vi "gfitsio-error-cluster-from-code.vi"(8 "error in (no error)":errorcluster, 11 "error code":i32) -> (0 "error out":errorcluster)   [LabVIEW 2015]
doc: "Converts an error code to an error cluster. If the CFITSIO error stack contains messages, these are placed in the \"source\" field of <B>error out</B>. If <B>error in</B> indicates that an error occurred before this VI or function ran, <B>error out</B> contains the same error information. Otherwise, it describes the error status corresponding to the <B>error code</B>."
uses:
  gfitsio.dll
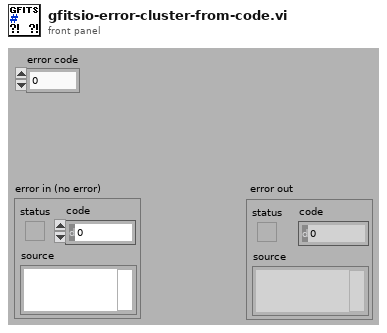
[diagram p1: front panel]
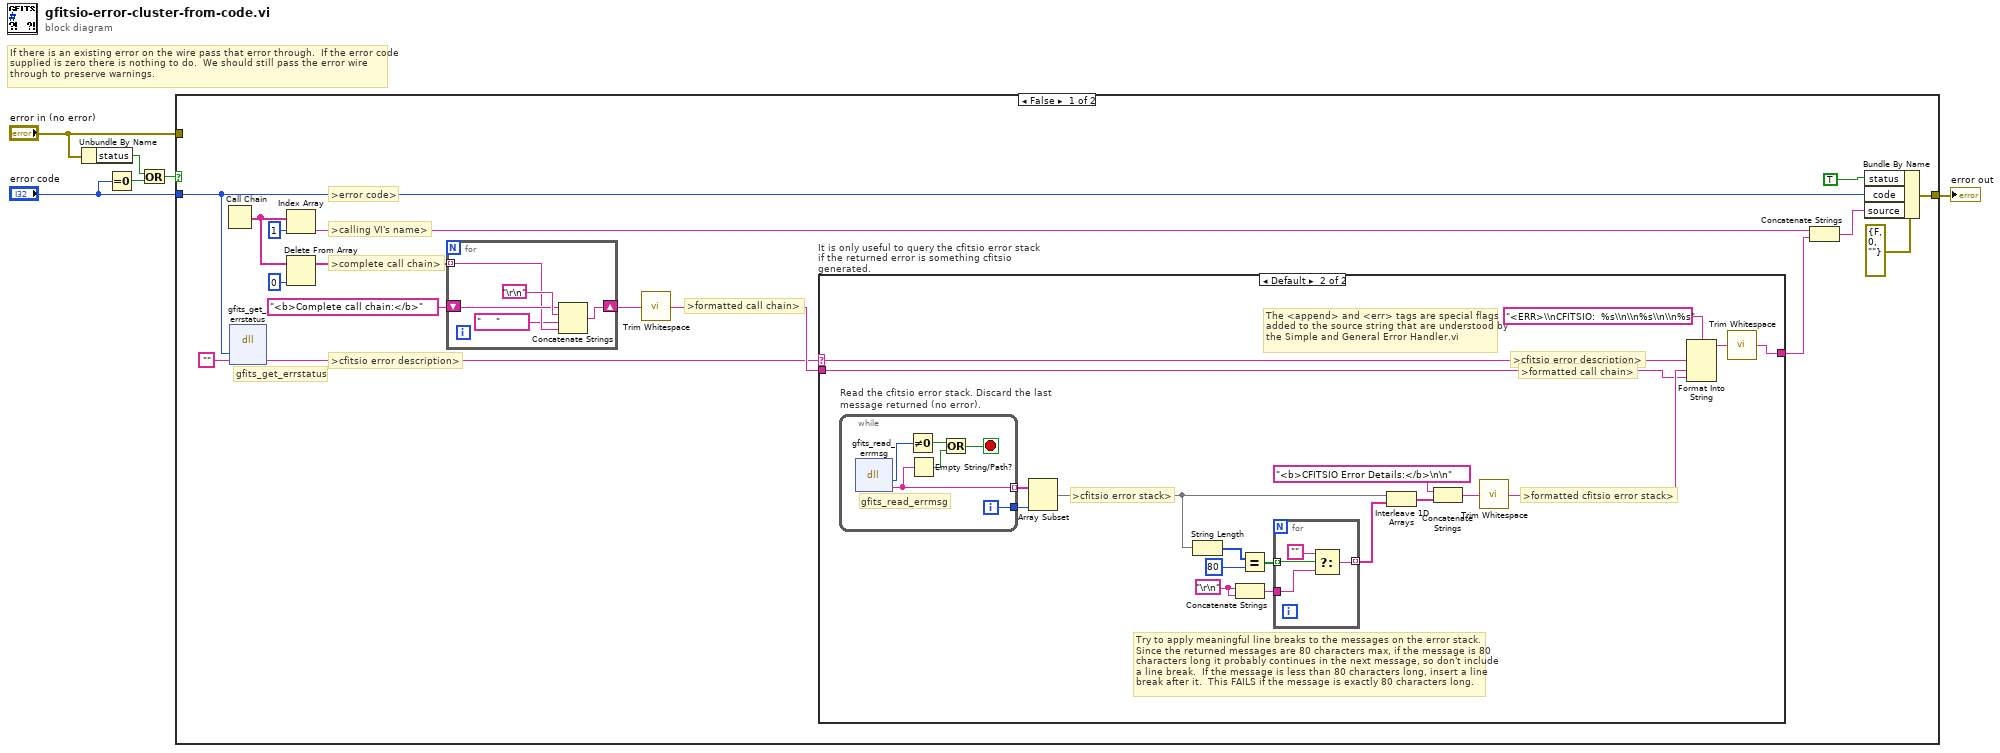
[diagram p0: block diagram]
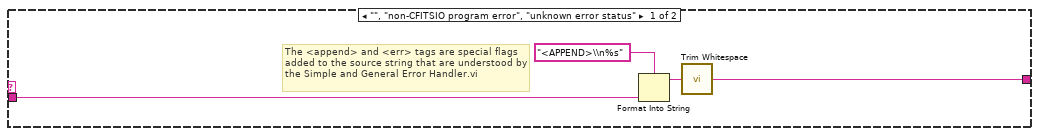
[diagram p2: hidden frame]
diagram:
  # "If there is an existing error on the wire pass that error through.  If the error code supplied is zero there is nothing to do.  We should still pass the error wire through to preserve warnings."
  n1 = Unbundle By Name("error in (no error)") -> ("status"=w4:bool)
  n2 = Equal To 0?(x="error code") -> (x = 0?=w5:bool)
  n3 = Or(x=w4, y=w5) -> (x .or. y?=w3:bool)
  n4 = case shown="False" w3 {
    tunnel: "error code" -> [w8 _]
    tunnel: "error in (no error)" -> [_ w60]
    tunnel: [w7 w60] -> w1
    frame False {
      # ">formatted call chain>"
      # ">cfitsio error description>"
      # "gfits_get_errstatus"
      # ">complete call chain>"
      # ">calling VI's name>"
      # ">error code>"
      n5 = Call Chain() -> (call chain=w18:string[])
      n6 = dll-call lib="C:/ALPHA GSCS/GSCS/Systems/SIcamera_Control/Quick_Look/gfitsio/gfitsio.dll" fn="gfits_get_errstatus"("status"=w8, "err_text"="") -> ("err_text"=w9:string)  [unwired: 5 in, 2 out]
      n7 = Index Array(array=w18, index=1) -> (element=w12:string)
      n8 = Delete From Array(array=w18, index=0) -> (array with subset deleted=w20:string[])  [unwired: 1 in, 1 out]
      n9 = for {
        tunnel: w20 -> [w56] mode=indexing
        shift-right: [w59] -> w11
        shift-left: "<b>Complete call chain:</b>" ("call chain header") -> [w57]
        n10 = Concatenate Strings(w57, "\r\n", "     ", w56) -> (w59:string)
      }
      n11 = call <vilib>:"Trim Whitespace.vi"("string"=w11) -> ("trimmed string"=w10:string)  [unwired: 1 in]
      n12 = case "It is only useful to query the cfitsio error stack if the returned error is something cfitsio generated." shown="Default" w9 {
        selector: w9 -> [_ w27]
        tunnel: [w24 w40] -> w13
        tunnel: w10 -> [w23 w28]
        frame "", "non-CFITSIO program error", "unknown error status" {
          # "The <append> and <err> tags are special flags added to the source string that are understood by the Simple and General Error Handler.vi"
          n13 = Format Into String(format string="<APPEND>\\n%s", w23) -> (resulting string=w26:string)  [unwired: 2 in, 1 out]
          n14 = call <vilib>:"Trim Whitespace.vi"("string"=w26) -> ("trimmed string"=w24:string)  [unwired: 1 in]
        }
        frame Default {
          w33 = "\r\n"
          # ">cfitsio error description>"
          # ">formatted call chain>"
          # "The <append> and <err> tags are special flags added to the source string that are understood by the Simple and General Error Handler.vi"
          # ">formatted cfitsio error stack>"
          # "Try to apply meaningful line breaks to the messages on the error stack.  Since the returned messages are 80 characters max, if the message is 80 characters long it probably continues in the next message, so don't include a line break.  If the message is less than 80 characters long, insert a line break after it.  This FAILS if the message is exactly 80 characters long."
          # ">cfitsio error stack>"
          n15 = while "Read the cfitsio error stack. Discard the last message returned (no error)." {
            tunnel: [w54] -> w44 mode=indexing
            tunnel: [w53] -> w43
            i -> [w53]
            stop <- w49 stop-if-true
            # "gfits_read_errmsg"
            n16 = dll-call lib="C:/ALPHA GSCS/GSCS/Systems/SIcamera_Control/Quick_Look/gfitsio/gfitsio.dll" fn="gfits_read_errmsg"() -> (w52:i32, "err_text"=w54:string)  [unwired: 4 in, 2 out]
            n17 = Not Equal To 0?(x=w52) -> (x != 0?=w50:bool)
            n18 = Empty String/Path?(string/path=w54) -> (empty?=w51:bool)
            n19 = Or(x=w50, y=w51) -> (x .or. y?=w49:bool)
          }
          n20 = Array Subset(array=w44, length=w43) -> (w31:string[])  [unwired: 1 in]
          n21 = String Length(string=w31) -> (length=w38:i32[])
          n22 = Concatenate Strings(w33, w33) -> (w32:string)
          n23 = Equal?(x=w38, y=80) -> (x = y?=w36:bool[])
          n24 = for {
            tunnel: w36 -> [w48] mode=indexing
            tunnel: [w46] -> w35 mode=indexing
            tunnel: w32 -> [w45]
            n25 = Select(t="", s=w48, f=w45) -> (s? t:f=w46:string)
          }
          n26 = Interleave 1D Arrays(w31, w35) -> (w34:string[])
          n27 = Concatenate Strings("<b>CFITSIO Error Details:</b>\n\n" ("string"), w34) -> (w30:string)
          n28 = call <vilib>:"Trim Whitespace.vi"("string"=w30) -> ("trimmed string"=w29:string)  [unwired: 1 in]
          n29 = Format Into String(format string="<ERR>\\nCFITSIO:  %s\\n\\n%s\\n\\n%s", w27, w29, w28) -> (resulting string=w42:string)  [unwired: 2 in, 1 out]
          n30 = call <vilib>:"Trim Whitespace.vi"("string"=w42) -> ("trimmed string"=w40:string)  [unwired: 1 in]
        }
      }
      n31 = Concatenate Strings(w12, w13) -> (w16:string)
      n32 = Bundle By Name(cluster=errorcluster {"status"=FALSE, "code"=0, "source"=""} ("error out"), "status"=TRUE, "code"=w8, "source"=w16) -> (w7:errorcluster)
    }
    frame True {
    }
  }
  "error out" <- w1
